vi "LWXPS_PositionerCompensationPostExcitationNotchModeFilterGet.vi"(0 "XPS Reference IN":refnum<k24>, 1 "Positioner Name":string, 4 "Notch Mode Number":i32, 5 "LabVIEW error IN":errorcluster) -> (12 "XPS Reference OUT":refnum<k24>, 13 "LabVIEW error OUT":errorcluster, 14 "Returned error code":i32, 15 "Resonance frequency":dbl, 16 "Anti-resonance frequency":dbl, 17 "Resonance damping factor":dbl, 18 "Anti-resonance damping factor":dbl, 19 "XPS Error String":string)   [LabVIEW 2014]
uses:
  D:/XPSQ8_LabView_Library/Development/Source/Dll/Newport.XPS.CommandInterface.dll
  Dll/Newport.XPS.CommandInterface.dll
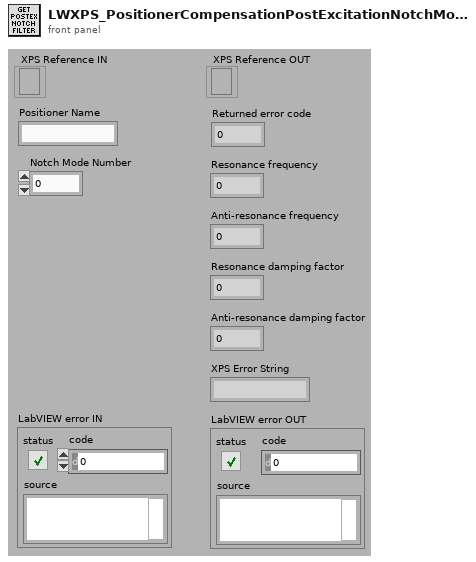
[diagram p1: front panel]
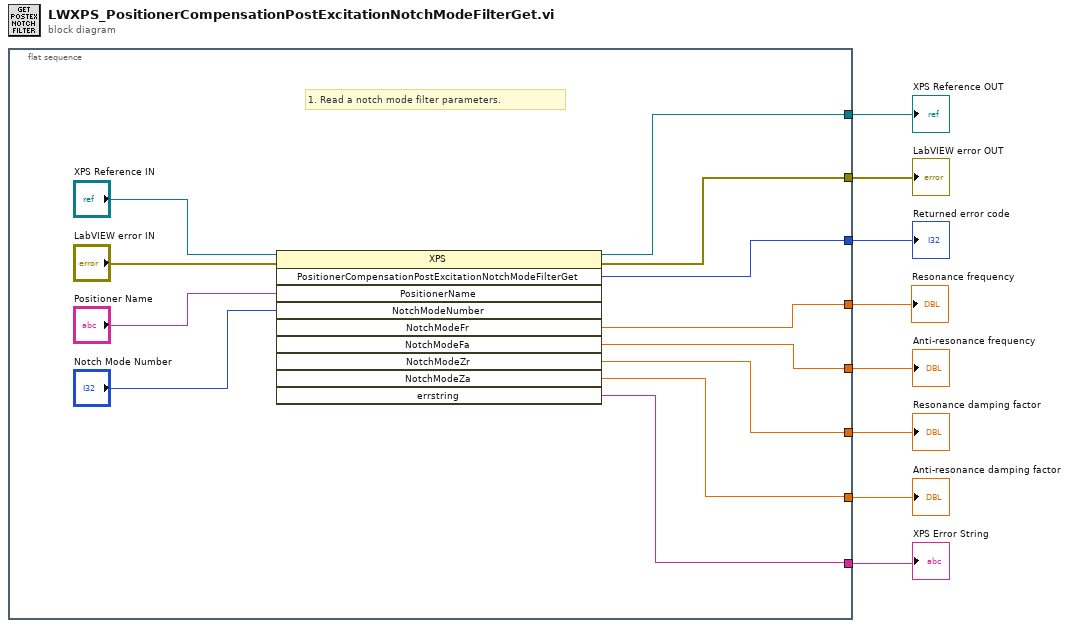
[diagram p0: block diagram]
diagram:
  n1 = flat-sequence {
    tunnel: [w18] -> w8
    tunnel: [w14] -> w7
    tunnel: [w19] -> w6
    tunnel: [w15] -> w5
    tunnel: [w12] -> w4
    tunnel: [w10] -> w3
    tunnel: [w11] -> w2
    tunnel: [w9] -> w1
    frame #0 {
      # "1. Read a notch mode filter parameters."
      n2 = invoke class="XPS" method="PositionerCompensationPostExcitationNotchModeFilterGet"(reference="XPS Reference IN", error in="LabVIEW error IN", "PositionerName"="Positioner Name", "NotchModeNumber"="Notch Mode Number") -> (reference out=w18:refnum<k24>, error out=w14:errorcluster, "PositionerCompensationPostExcitationNotchModeFilterGet"=w19:i32, "NotchModeFr"=w15:dbl, "NotchModeFa"=w12:dbl, "NotchModeZr"=w10:dbl, "NotchModeZa"=w11:dbl, "errstring"=w9:string)  [unwired: 6 in, 2 out]
    }
  }
  "XPS Error String" <- w1
  "XPS Reference OUT" <- w8
  "LabVIEW error OUT" <- w7
  "Returned error code" <- w6
  "Resonance frequency" <- w5
  "Anti-resonance frequency" <- w4
  "Resonance damping factor" <- w3
  "Anti-resonance damping factor" <- w2
